vi "findDistanceToBreak.vi"(0 "Game in":refnum<class "Game.lvclass">, 1 "dist_robot_target":dbl, 5 "est_vel":dbl format="%#_13g", 9 "desired_vel":dbl, 11 "error in (no error)":errorcluster, 12 "v_sample":dbl, 13 "robotModel":dbl[][](array[numeric]), 14 "delta":dbl) -> (4 "Game out":refnum<class "Game.lvclass">, 6 "vel":dbl, 8 "DistanceToBreak":dbl, 10 "Robot Model":T1, 15 "error out":errorcluster)   [LabVIEW 2023, in "Game.lvclass"]
uses:
  Game.lvclass
  Controls/RobotModel.ctl
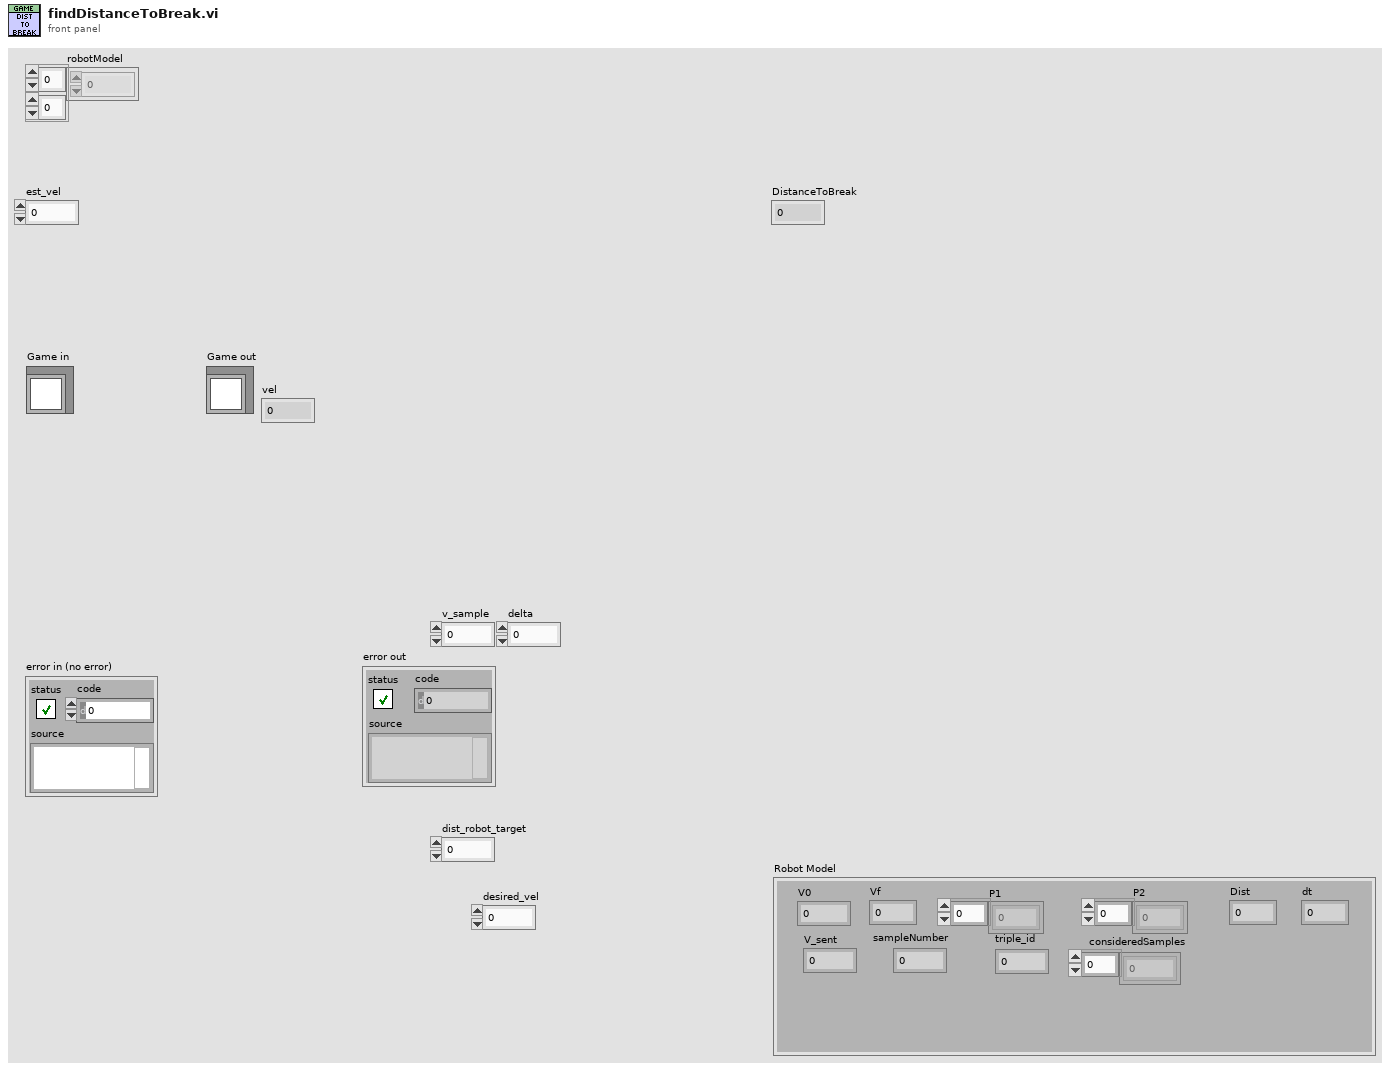
[diagram p1: front panel]
types:
  T1 = typedef "RobotModel.ctl" = cluster{"V0":dbl, "Vf":dbl, "Dist":dbl, "dt":dbl, "P1":dbl[], "P2":dbl[], "V_sent":dbl, "sampleNumber":i32, "triple_id":i32, "consideredSamples":dbl[]}
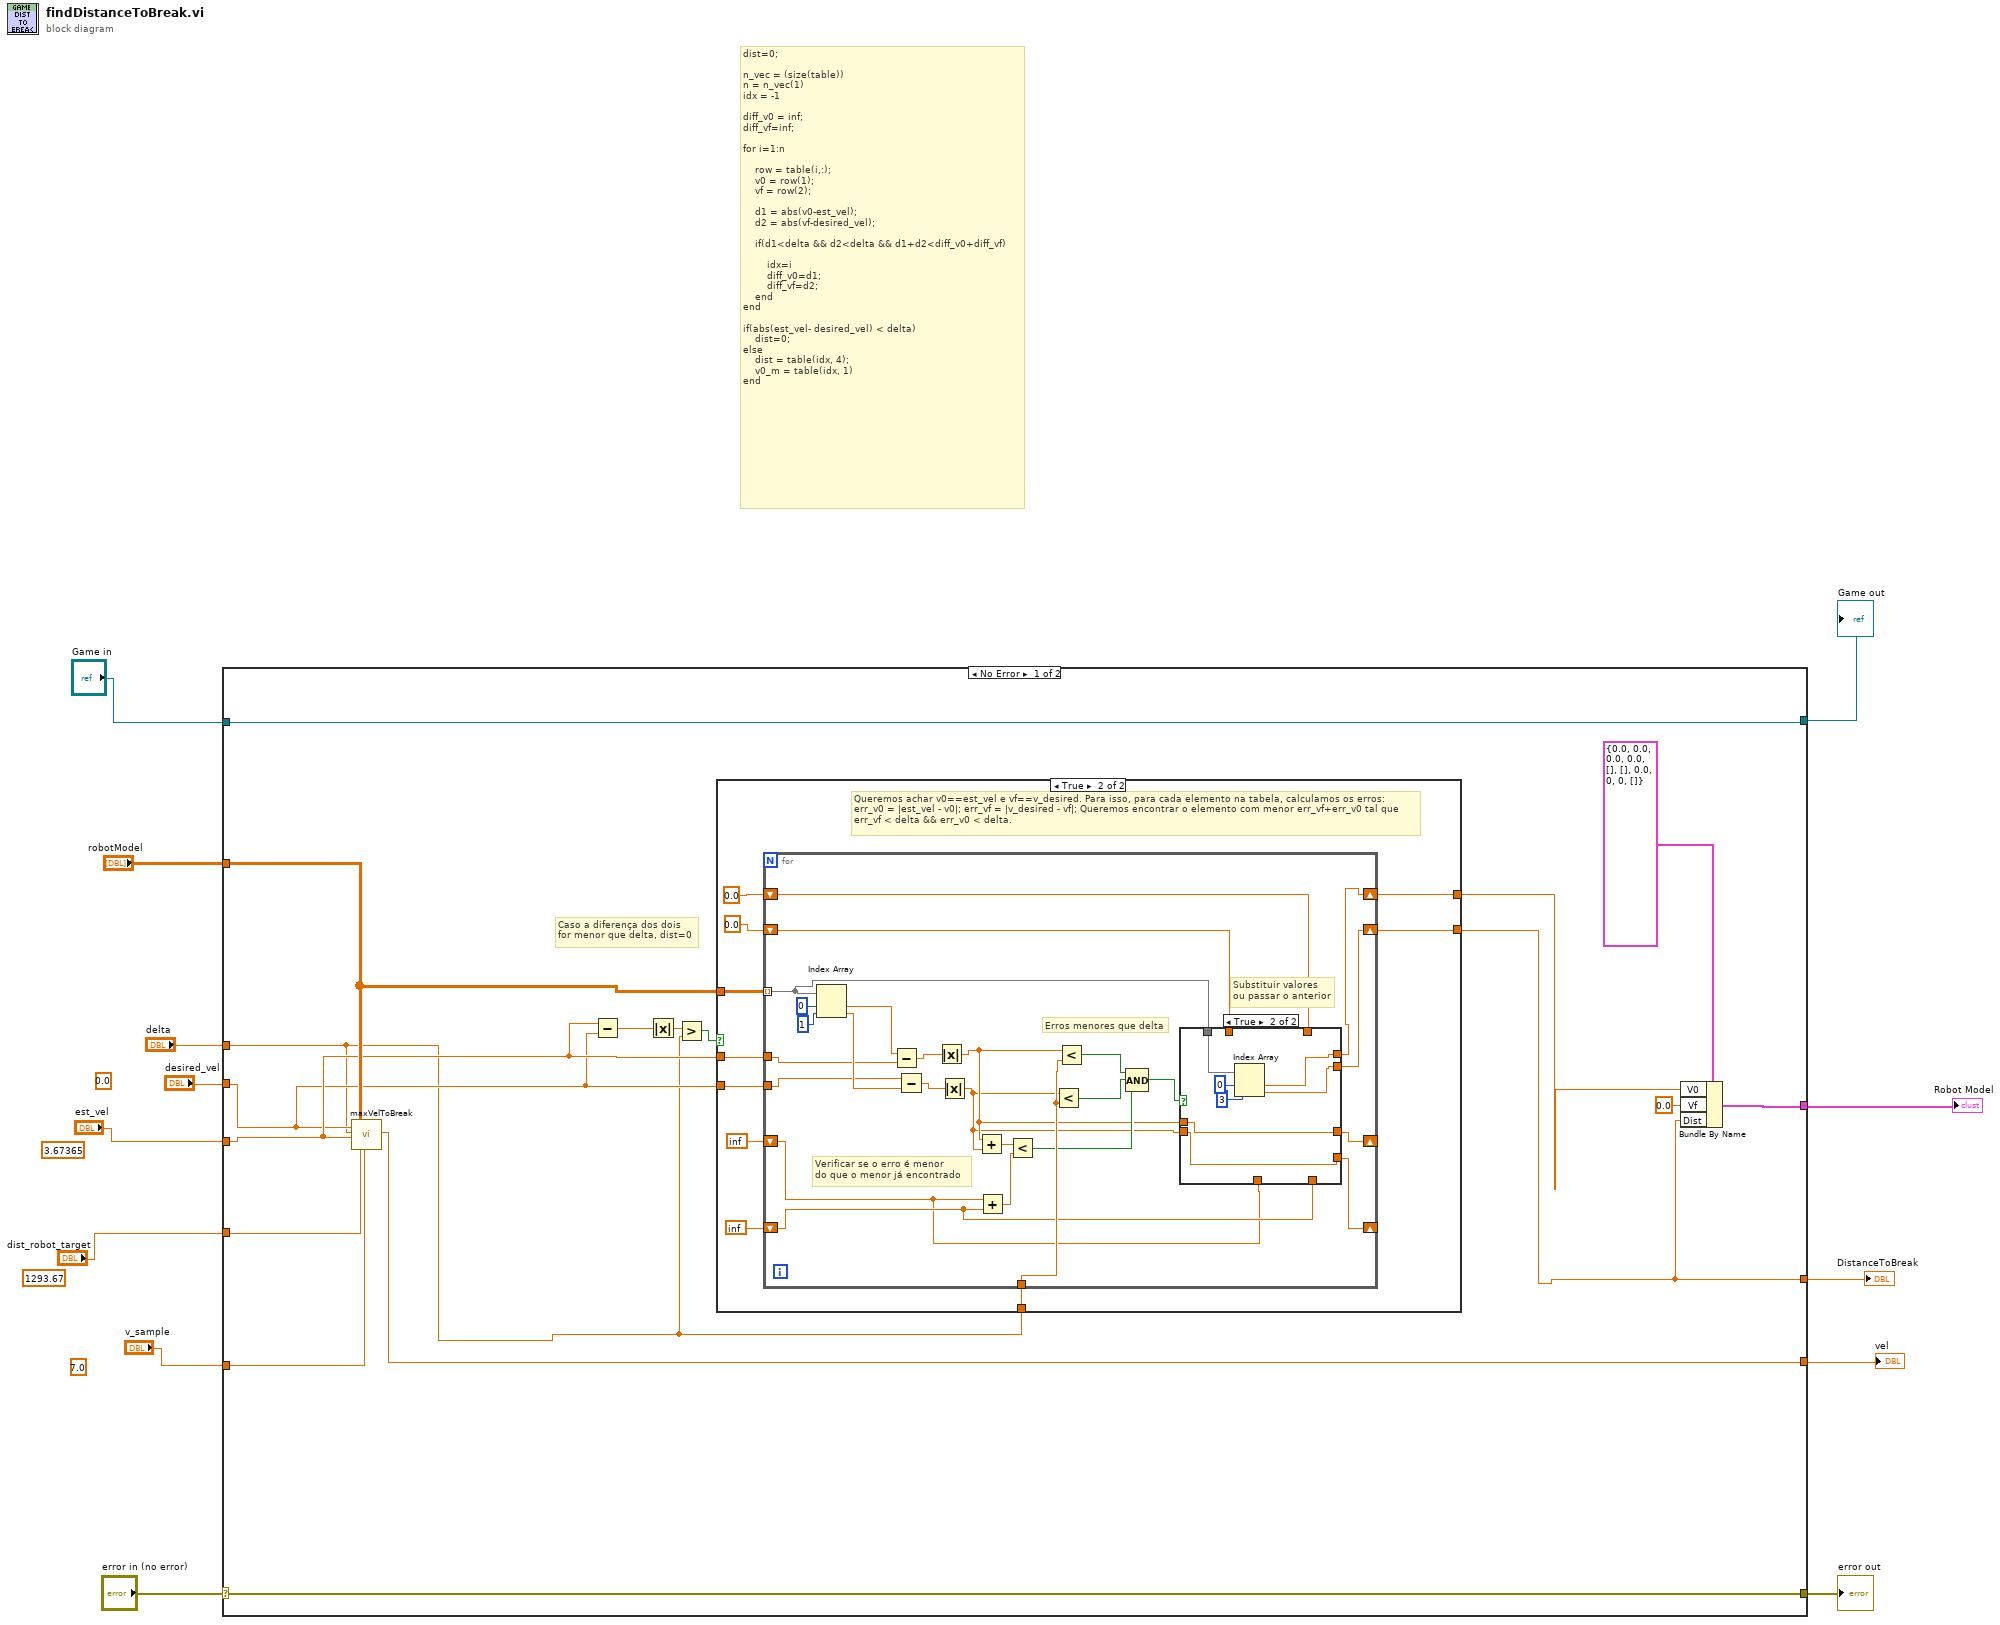
[diagram p0: block diagram]
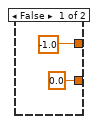
[diagram p2: hidden frame]
diagram:
  (unwired) 0.0 ("desired_vel")
  (unwired) 7.0 ("v_sample")
  (unwired) 1293.67
  (unwired) 3.67365
  # "dist=0;\n\nn_vec = (size(table))\nn = n_vec(1)\nidx = -1\n\ndiff_v0 = inf;\ndiff_vf=inf;\n\nfor i=1:n\n\n    row = table(i,:);\n    v0 = row(1);\n    vf = row(2);\n\n    d1 = abs(v0-est_vel);\n    d2 = abs(vf-desired_vel);\n\n    if(d1<delta && d2<delta && d1+d2<diff_v0+diff_vf)\n\n        idx=i\n        diff_v0=d1;\n        diff_vf=d2;\n    end\nend\n\nif(abs(est_vel- desired_vel) < delta)\n    dist=0;\nelse\n    dist = table(idx, 4);\n    v0_m = table(idx, 1)\nend"
  n1 = case shown="No Error" "error in (no error)" {
    selector: "error in (no error)" -> [w29 w81]
    tunnel: [w29 w81] -> w12
    tunnel: [w30 w80] -> w10
    tunnel: "Game in" -> [w30 w80]
    tunnel: "est_vel" -> [w20 _]
    tunnel: "robotModel" -> [w21 _]
    tunnel: "desired_vel" -> [w19 _]
    tunnel: "v_sample" -> [w25 _]
    tunnel: "delta" -> [w18 _]
    tunnel: [w28 _] -> w9
    tunnel: "dist_robot_target" -> [w26 _]
    tunnel: [w24 _] -> w8
    tunnel: [w17 _] -> w7
    frame No Error {
      # "Caso a diferença dos dois\nfor menor que delta, dist=0"
      n2 = call "maxVelToBreak.vi"("desired_vel"=w19, "delta"=w18, "est_vel"=w20, "array"=w21, "dist"=w26, "v_max"=w25) -> ("vel"=w24:dbl)  [unwired: 11 in, 2 out]
      n3 = Subtract(x=w20, y=w19) -> (x-y=w16:dbl)
      n4 = Absolute Value(x=w16) -> (abs(x)=w15:dbl)
      n5 = Greater?(x=w15, y=w18) -> (0:w14:bool)
      n6 = case shown="True" w14 {
        tunnel: w21 -> [_ w42]
        tunnel: w20 -> [_ w41]
        tunnel: w19 -> [_ w40]
        tunnel: w18 -> [_ w39]
        tunnel: [-1.0 w36] -> w23
        tunnel: [0.0 w35] -> w17
        frame False {
        }
        frame True {
          # "Queremos achar v0==est_vel e vf==v_desired. Para isso, para cada elemento na tabela, calculamos os erros:\nerr_v0 = |est_vel - v0|; err_vf = |v_desired - vf|; Queremos encontrar o elemento com menor err_vf+err_v0 tal que\nerr_vf < delta && err_v0 < delta."
          n7 = for {
            tunnel: w42 -> [w47] mode=indexing
            tunnel: w41 -> [w63]
            tunnel: w40 -> [w65]
            tunnel: w39 -> [w60]
            shift-right: [w51] -> _
            shift-left: inf -> [w48]
            shift-right: [w50] -> _
            shift-left: inf -> [w49]
            shift-right: [w44] -> w36
            shift-left: 0.0 -> [w45]
            shift-right: [w43] -> w35
            shift-left: 0.0 -> [w46]
            # "Substituir valores\nou passar o anterior"
            # "Verificar se o erro é menor\ndo que o menor já encontrado"
            # "Erros menores que delta"
            n8 = Index Array(array=w47, index #1=0 ("index"), index #2=1 ("index")) -> (element #1=w64:dbl, element #2=w66:dbl)
            n9 = Subtract(x=w64, y=w63) -> (x-y=w62:dbl)
            n10 = Subtract(x=w65, y=w66) -> (x-y=w61:dbl)
            n11 = Absolute Value(x=w62) -> (abs(x)=w53:dbl)
            n12 = Absolute Value(x=w61) -> (abs(x)=w52:dbl)
            n13 = Add(x=w53, y=w52) -> (x+y=w59:dbl)
            n14 = Add(x=w48, y=w49) -> (x+y=w58:dbl)
            n15 = Less?(x=w59, y=w58) -> (x < y?=w55:bool)
            n16 = Less?(x=w52, y=w60) -> (x < y?=w56:bool)
            n17 = Less?(x=w53, y=w60) -> (x < y?=w57:bool)
            n18 = Compound Arithmetic op=AND(w57, w56, w55) -> (w54:bool)
            n19 = case shown="True" w54 {
              tunnel: w53 -> [_ w79]
              tunnel: w52 -> [_ w78]
              tunnel: [w71 w79] -> w51
              tunnel: [w72 w78] -> w50
              tunnel: w49 -> [w72 _]
              tunnel: w48 -> [w71 _]
              tunnel: w47 -> [_ w77]
              tunnel: w46 -> [w69 _]
              tunnel: w45 -> [w70 _]
              tunnel: [w70 w74] -> w44
              tunnel: [w69 w73] -> w43
              frame False {
              }
              frame True {
                n20 = Index Array(array=w77, index #1=0 ("index"), index #2=3 ("index")) -> (element #1=w74:dbl, element #2=w73:dbl)
              }
            }
          }
        }
      }
      n21 = Bundle By Name(cluster=T1 {"V0"=0.0, "Vf"=0.0, "Dist"=0.0, "dt"=0.0, "P1"=[], "P2"=[], "V_sent"=0.0, "sampleNumber"=0, "triple_id"=0, "consideredSamples"=[]} ("Robot Model"), "V0"=w23, "Vf"=0.0, "Dist"=w17) -> (w28:T1)
    }
    frame Error {
    }
  }
  "error out" <- w12
  "Game out" <- w10
  "DistanceToBreak" <- w7
  "Robot Model" <- w9
  "vel" <- w8
